vi "Get Project MyComputer.vi"(8 "error in":errorcluster) -> (0 "error out":errorcluster, 3 "My Computer":refnum<vi>)   [LabVIEW 2021, in "Missing in Project.lvclass"]
doc: "Returns the MyComputer reference to the project."
uses:
  Missing in Project.lvclass
  Missing in Project.lvclass/Missing in Project.ctl
panel:
  out "project path":path
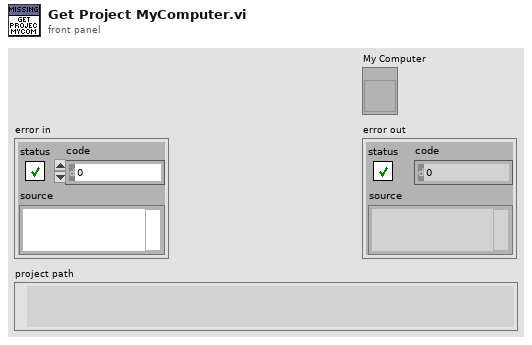
[diagram p1: front panel]
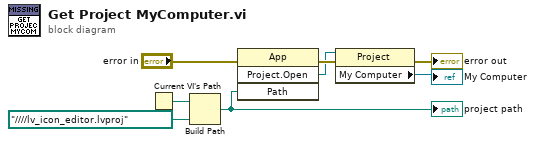
[diagram p0: block diagram]
diagram:
  n1 = Current VI's Path() -> (path=w4:path)
  n2 = Build Path(base path=w4, name or relative path=path "../../../../lv_icon_editor.lvproj") -> (appended path=w2:path)
  "project path" <- w2
  n3 = invoke class="App" method="Project.Open"(error in="error in", "Path"=w2) -> (error out=w8:errorcluster, "Project:Open"=w3:refnum<vi>)  [unwired: 2 in, 2 out]
  n4 = property class="Project"(reference=w3, error in=w8) -> (error out=→"error out":errorcluster, "My Computer"=→"My Computer":refnum<vi>)  [unwired: 1 out]
